vi "HexStringToBinaryString.vi"(11 "Hex String":string) -> (3 "Binary String":string)   [LabVIEW 2014]
panel:
  out "Array":string[](array[string])
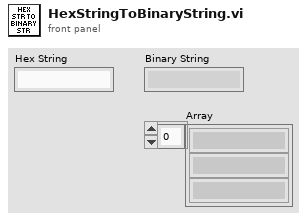
[diagram p1: front panel]
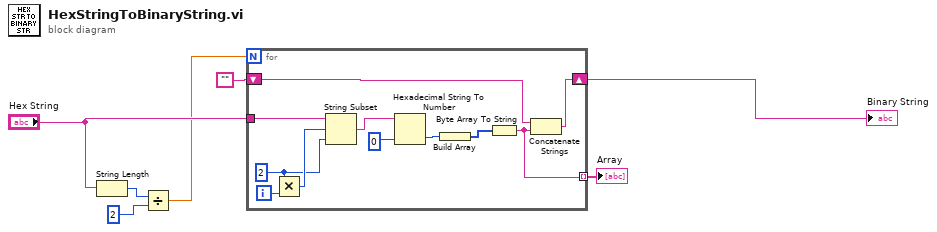
[diagram p0: block diagram]
diagram:
  n1 = String Length(string="Hex String") -> (length=w1:i32)
  n2 = Divide(x=w1, y=2) -> (x/y=w3:dbl)
  n3 = for {
    N: w3 -> [_]
    tunnel: "Hex String" -> [w11]
    shift-right: [w14] -> w7
    shift-left: "" ("string") -> [w13]
    tunnel: [w12] -> w5 mode=indexing
    i -> [w15]
    w8 = 2 ("x")
    n4 = Multiply(x=w8, y=w15) -> (x*y=w10:i32)
    n5 = String Subset(string=w11, offset (0)=w10, length (rest)=w8) -> (substring=w9:string)
    n6 = Hexadecimal String To Number(string=w9, default (0uL)=u8 0 ("default (0 U32)")) -> (number=w18:u8)  [unwired: 1 in, 1 out]
    n7 = Build Array(w18) -> (w17:u8[])
    n8 = Byte Array To String(unsigned byte array=w17) -> (string=w12:string)
    n9 = Concatenate Strings(w13, w12) -> (w14:string)
  }
  "Array" <- w5
  "Binary String" <- w7
